vi "NanotecSMCPDDriver.ID query.vi"(0 "VISA resource name":refnum<visa-resource-name>, 1 "contollerID":i32=-1, 5 "error in (no error)":errorcluster) -> (14 "VISA resource name out":refnum<visa-resource-name>, 15 "contollerID out":i32=-1, 16 "hardwareType":T1, 17 "hardwareTypeString":string, 19 "error out":errorcluster)   [LabVIEW 2014, in "NanotecSMCPDDriver.lvlib"]
doc: "Queries the current instrument mode (a real ID like serial number is not supported)"
uses:
  NanotecSMCPDDriver.lvlib
  Private/NanotecSMCPDDriver.hardware types.ctl
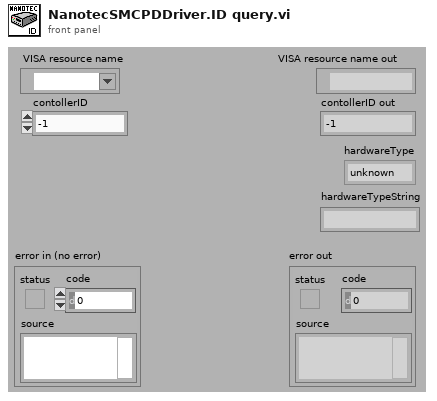
[diagram p1: front panel]
types:
  T1 = typedef "NanotecSMCPDDriver.lvlib/NanotecSMCPDDriver.hardware types.ctl" = enum16{"unknown", "PD4", "PD4Ic", "PD2Ic", "SMCI32", "SMCI47"}
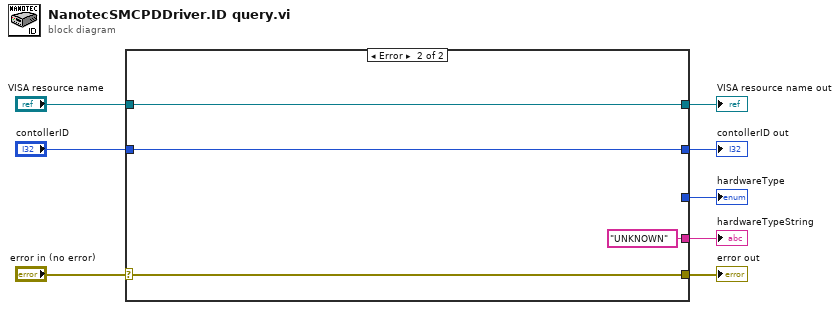
[diagram p0: block diagram]
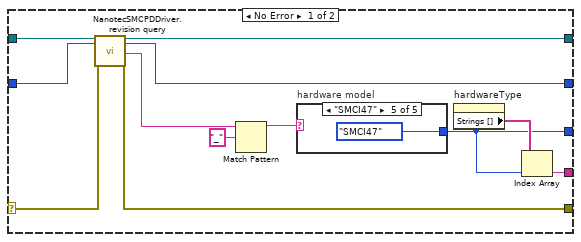
[diagram p2: hidden frame]
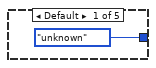
[diagram p3: hidden frame]
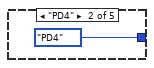
[diagram p4: hidden frame]
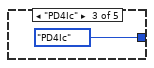
[diagram p5: hidden frame]
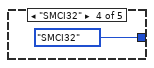
[diagram p6: hidden frame]
diagram:
  n1 = case shown="Error" "error in (no error)" {
    selector: "error in (no error)" -> [w18 w27]
    tunnel: [w17 w29] -> w8
    tunnel: [w15 w27] -> w7
    tunnel: "VISA resource name" -> [w20 w29]
    tunnel: "contollerID" -> [w19 w28]
    tunnel: [w16 w28] -> w4
    tunnel: [w9 _] -> w2
    tunnel: [w10 "UNKNOWN"] -> w1
    frame No Error {
      n2 = call "NanotecSMCPDDriver.revision query.vi"("VISA resource name"=w20, "contollerID"=w19, "error in (no error)"=w18) -> ("VISA resource name out"=w17:refnum<visa-resource-name>, "contollerID out"=w16:i32, "Instrument Firmware Revision"=w14:string, "error out"=w15:errorcluster)  [unwired: 12 in, 1 out]
      n3 = Match Pattern(string=w14, regular expression="_") -> (before substring=w12:string)  [unwired: 1 in, 3 out]
      n4 = case "hardware model" shown="\"SMCI47\"" w12 {
        tunnel: [NanotecSMCPDDriver.hardware_types."unknown" ("hardwareType") NanotecSMCPDDriver.hardware_types."PD4" ("hardwareType") NanotecSMCPDDriver.hardware_types."PD4Ic" ("hardwareType") NanotecSMCPDDriver.hardware_types."SMCI32" ("hardwareType") NanotecSMCPDDriver.hardware_types."SMCI47" ("hardwareType")] -> w9
        frame Default {
        }
        frame "PD4" {
        }
        frame "PD4Ic" {
        }
        frame "SMCI32" {
        }
        frame "SMCI47" {
        }
      }
      n5 = property on="hardwareType" class="Enum (strict)"() -> ("Strings []"=w11:string[])  [unwired: 2 in, 2 out]
      n6 = Index Array(array=w11, index=w9) -> (element=w10:string)
    }
    frame Error {
    }
  }
  "VISA resource name out" <- w8
  "error out" <- w7
  "contollerID out" <- w4
  "hardwareType" <- w2
  "hardwareTypeString" <- w1
